vi "Obtain View.vi"(0 "Serial port assistant view in":refnum<class "Serial port assistant view.lvclass">, 11 "error in (no error)":errorcluster) -> (4 "Serial port assistant view out":refnum<class "Serial port assistant view.lvclass">, 15 "error out":errorcluster)   [LabVIEW 2022 SP3, in "Serial port assistant view.lvlib" / "Serial port assistant view.lvclass"]
uses:
  Serial port assistant view.lvclass
  serial port list--type.ctl
  serial port status--type.ctl
  data has been sent--type.ctl
  data has been received--type.ctl
  forced exit--type.ctl
  Serial port assistant view.lvclass/Serial port assistant view.ctl
  user interface.vi
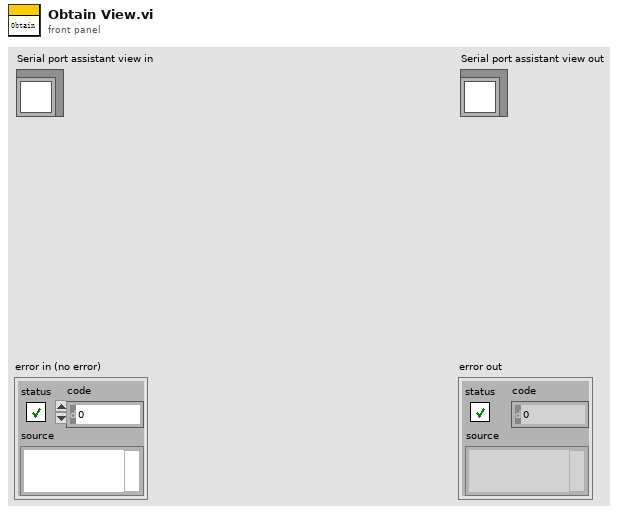
[diagram p1: front panel]
types:
  T1 = typedef "Serial port assistant view.lvlib/Serial port assistant view.lvclass/forced exit--type.ctl" = cluster{"message":string}
  T2 = enum32{"Invalid", "Standard", "Closed", "Hidden", "Minimized", "Maximized"}
  T3 = typedef "Serial port assistant view.lvlib/Serial port assistant view.lvclass/data has been received--type.ctl" = cluster{"receive time":string, "data has been received":string}
  T4 = typedef "Serial port assistant view.lvlib/Serial port assistant view.lvclass/data has been sent--type.ctl" = cluster{"send time":string, "data has been sent":string}
  T5 = typedef "Serial port assistant view.lvlib/Serial port assistant view.lvclass/serial port status--type.ctl" = cluster{"serial port":string, "baud rate":u32, "data bits":u16, "stop bits":u16, "parity":u16, "open":bool}
  T6 = typedef "Serial port assistant view.lvlib/Serial port assistant view.lvclass/serial port list--type.ctl" = cluster{"serial port list":string[]}
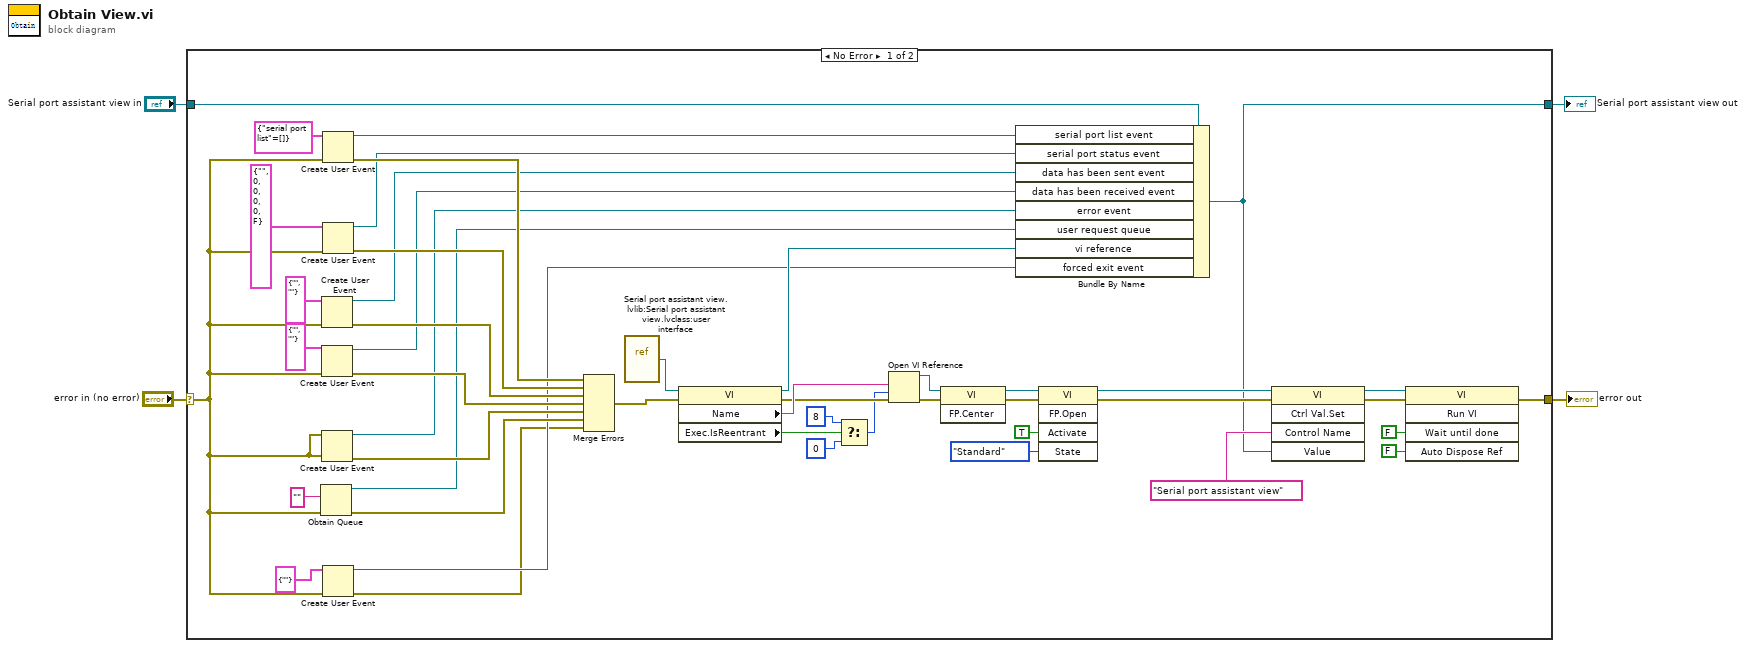
[diagram p0: block diagram]
diagram:
  n1 = case shown="No Error" "error in (no error)" {
    selector: "error in (no error)" -> [w8 w52]
    tunnel: [w30 w52] -> w3
    tunnel: "Serial port assistant view in" -> [w49 w51]
    tunnel: [w21 w51] -> w1
    frame No Error {
      n2 = Obtain Queue(element data type="", error in (no error)=w8) -> (queue out=w10:refnum<queue>, error out=w15:errorcluster)  [unwired: 3 in, 1 out]
      n3 = Create User Event(user event datatype=T4 {"send time"="", "data has been sent"=""} ("data has been sent"), error in=w8) -> (user event=w12:refnum<user-event>, error out=w18:errorcluster)
      n4 = Create User Event(user event datatype=T3 {"receive time"="", "data has been received"=""} ("data has been received"), error in=w8) -> (user event=w11:refnum<user-event>, error out=w17:errorcluster)
      n5 = Create User Event(user event datatype=w8, error in=w8) -> (user event=w9:refnum<user-event>, error out=w16:errorcluster)
      n6 = Create User Event(user event datatype=T6 {"serial port list"=[]} ("serial port list"), error in=w8) -> (user event=w48:refnum<user-event>, error out=w20:errorcluster)
      n7 = Create User Event(user event datatype=T5 {"serial port"="", "baud rate"=0, "data bits"=0, "stop bits"=0, "parity"=0, "open"=FALSE} ("serial port status"), error in=w8) -> (user event=w13:refnum<user-event>, error out=w19:errorcluster)
      n8 = Create User Event(user event datatype=T1 {"message"=""} ("forced exit"), error in=w8) -> (user event=w6:refnum<user-event>, error out=w5:errorcluster)
      n9 = Merge Errors(w20, w19, w18, w17, w16, w15, w5) -> (w14:errorcluster)
      n10 = vi-ref "Serial port assistant view.lvlib:Serial port assistant view.lvclass:user interface.vi"() -> (w44:refnum<vi>)
      n11 = property class="VI"(reference=w44, error in=w14) -> (reference out=w27:refnum<vi>, error out=w41:errorcluster, "Name"=w43:string, "Exec.IsReentrant"=w42:bool)
      n12 = Select(t=8 ("options"), s=w42, f=0 ("options")) -> (s? t:f=w38:i32)
      n13 = Open VI Reference(vi path=w43, options=w38, error in (no error)=w41) -> (vi reference=w29:refnum<vi>, error out=w36:errorcluster)  [unwired: 3 in]
      n14 = invoke class="VI" method="FP.Center"(reference=w29, error in=w36) -> (reference out=w37:refnum<vi>, error out=w35:errorcluster)  [unwired: 1 in, 1 out]
      n15 = Bundle By Name(cluster=w49, "serial port list event"=w48, "serial port status event"=w13, "data has been sent event"=w12, "data has been received event"=w11, "error event"=w9, "user request queue"=w10, "vi reference"=w27, "forced exit event"=w6) -> (w21:refnum<class "Serial port assistant view.lvclass">)
      n16 = invoke class="VI" method="FP.Open"(reference=w37, error in=w35, "Activate"=TRUE ("Activate?"), "State"=T2."Standard") -> (reference out=w26:refnum<vi>, error out=w25:errorcluster)  [unwired: 1 in, 3 out]
      n17 = invoke class="VI" method="Ctrl Val.Set"(reference=w26, error in=w25, "Control Name"="Serial port assistant view", "Value"=w21) -> (reference out=w24:refnum<vi>, error out=w23:errorcluster)  [unwired: 1 in, 3 out]
      n18 = invoke class="VI" method="Run VI"(reference=w24, error in=w23, "Wait until done"=FALSE ("Wait Until Done"), "Auto Dispose Ref"=FALSE ("Auto Dispose Reference")) -> (error out=w30:errorcluster)  [unwired: 1 in, 4 out]
    }
    frame Error {
    }
  }
  "error out" <- w3
  "Serial port assistant view out" <- w1
